vi "_io_read_long_data_chunked_timeout.vi"(4 "Simulation read buffer (\"Simulation\")":string="Simulation", 5 "Timeout for chunked touts (-1: No chunked touts)":i32=-1, 6 "Block Logging (F)":bool, 7 "Block Delay Before Read (F)":bool, 8 "error in":errorcluster caption="error in (no error)", 9 "Trim Response End":bool=TRUE, 10 "Max segment read bytes count (65536)":u32=65536, 11 "VISA resource name":refnum<visa-resource-name>) -> (0 "error out":errorcluster, 1 "TimedOut":bool, 2 "Read buffer":string, 3 "VISA resource name out":refnum<visa-resource-name>)   [LabVIEW 2022 SP3, in "hmp4000_rsidr_core.lvlib"]
doc: "Reads data of unlimited size with chunked VISA timeout - use it for long timeouts, where setting the VISA timeout so high would make the LabVIEW application unresponsive until VISA returns from VISA Read function. The maximum VISA Timeout in this method is 10 seconds, and cumulatively goes up to entered timeout value."
uses:
  hmp4000_rsidr_core.lvlib
  type_Error_Codes.ctl
  type_AdditionalFlag_Bits.ctl
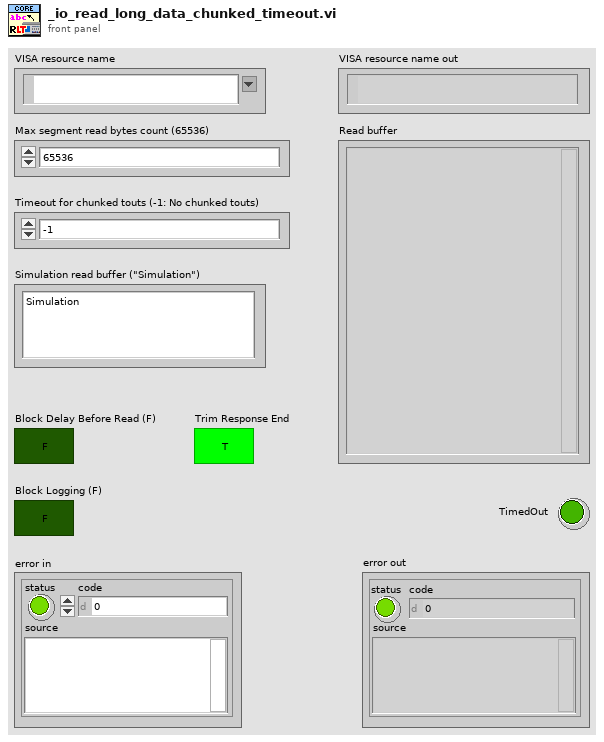
[diagram p1: front panel]
types:
  T1 = typedef "hmp4000_rsidr_core.lvlib/type_AdditionalFlag_Bits.ctl" = enum16{"Send LF after Bin Block", "Junk read with io_clear_buffers.vi", "io_clear_buffers: viClear()", "io_clear_buffers: viFlush()", "<NotUsed1>", "Allow Dbl & Int Bin/Ascii read", "*OPC? in check_instrument_error.vi", "<NotUsed2>", "Smart Enum Matching", "Less Strict RepCaps check", "AssureResponseEndWithLF"}
  T2 = typedef "hmp4000_rsidr_core.lvlib/type_Error_Codes.ctl" = enum16{"No_error", "VISA_err_ResourceNotFound", "VISA_err_Timeout", "VISA_warn_MoreDataAvailable", "RS_err_MissingCallback", "RS_err_InvalidAttribute", "RS_err_InvalidValue", "RS_err_UnknownResource", "RS_err_AlreadyInitialized", "RS_err_InstrumentStatus", "RS_err_BadRepCapName", "RS_err_TypesMismatch", "RS_err_ValueNotSupported", "RS_err_InvalidRngTable", "RS_err_IDqueryFail", "RS_err_UnexpResponse", "VISA_warn_ConfigNotLoaded", "RS_err_AttributeNotReadable", "RS_err_AttributeNotWritable", "RS_err_InstrumentType", "RS_err_InstrumentOption", "VISA_err_InvalidSize", "RS_err_ReliabilityIndicator", "VISA_warn_UnknownStatus", "VISA_warn_TermCharRead", "VISA_err_IO_error", "RS_err_FunctionNotSupported", "VISA_warn_QueueEmpty"}
  T3 = typedef "hmp4000_rsidr_core.lvlib/type_Session_Data.ctl" = cluster{"IDN string":string, "Instrument FW":string, "Instr type":string, "Instr type for err. msg.":string, "Installed Options":string[], "Ignore Error Messages":string, "Logging params":variant, "OPC Timeout":i32, "VISA Timeout":i32, "STB Poll VISA Timeout":i32, "Additional Flags":i32, "Wait Before Read":i32, "Wait Before Write":i32, "Option String Flags":i32, "IO Segment Size":i64, "VISA Access Mode":T4, "Interface Type":T5, "OPC Wait Mode":T6, "Bin Float Number  Format":T7, "Bin Integer Number Format":T8, "Simulate":bool, "VXIcapable":bool, "Duplicate Session":bool, "Add LF to Write":bool, "Logging":bool, "Fast Sweep":bool, "Query Instrument Status":bool, "Check Range":bool, "Check Options":bool}
  T4 = typedef "hmp4000_rsidr_core.lvlib/type_VisaAccessMode.ctl" = u16
  T5 = typedef "hmp4000_rsidr_core.lvlib/type_InterfaceType.ctl" = enum16{"Unknown", "GPIB", "VXI", "GPIB_VXI", "ASRL", "PXI", "TCPIP", "USB", "SOCKET"}
  T6 = typedef "hmp4000_rsidr_core.lvlib/type_OPC_Wait_Mode.ctl" = enum16{"STBpolling", "STBpollingSlow", "STBpollingSuperSlow", "ServiceRequest", "OPCquery"}
  T7 = typedef "hmp4000_rsidr_core.lvlib/type_Binary_Float_Number_Format.ctl" = enum16{"Float_4_Bytes_Swapped", "Float_4_Bytes", "Double_8_Bytes_Swapped", "Double_8_Bytes"}
  T8 = typedef "hmp4000_rsidr_core.lvlib/type_Binary_Integer_Number_Format.ctl" = enum16{"Int32_4_Bytes_Swapped", "Int32_4 Bytes", "Int16_2_Bytes_Swapped", "Int16_2_Bytes"}
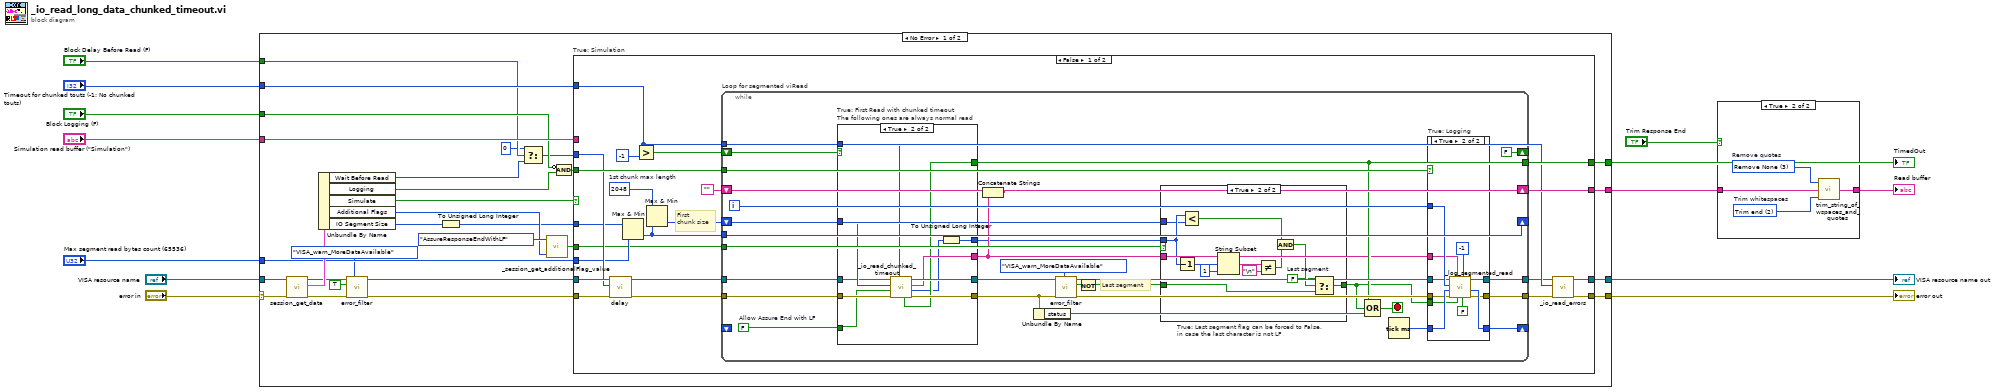
[diagram p0: block diagram]
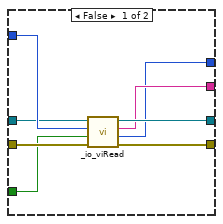
[diagram p5: hidden frame]
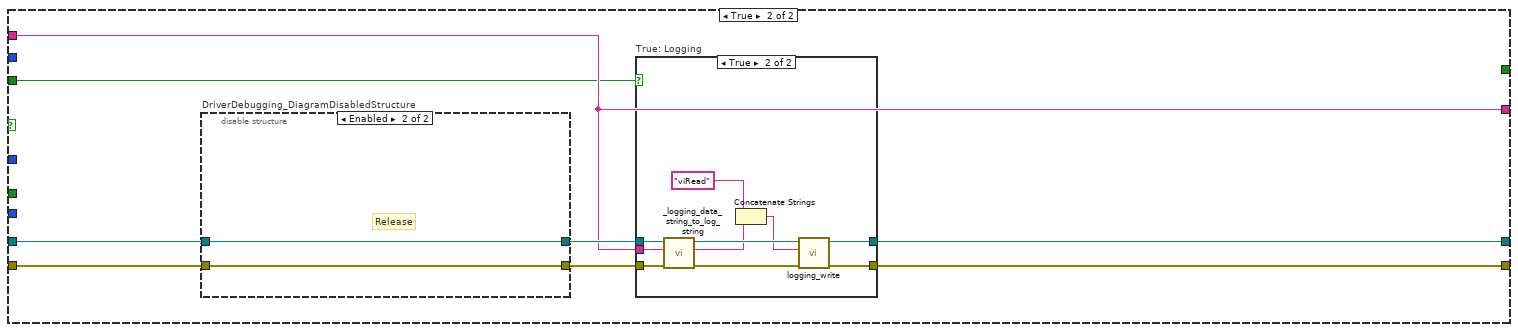
[diagram p6: hidden frame]
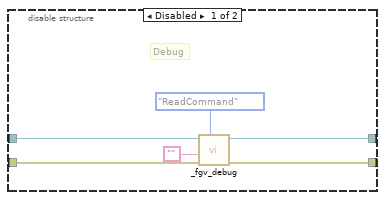
[diagram p8: hidden frame]
diagram:
  n1 = case shown="No Error" "error in" {
    selector: "error in" -> [w42 w171]
    tunnel: [w28 w171] -> w10
    tunnel: "Max segment read bytes count (65536)" -> [w38 _]
    tunnel: [w39 _] -> w2
    tunnel: "VISA resource name" -> [w41 w170]
    tunnel: [w27 w170] -> w9
    tunnel: "Simulation read buffer (\"Simulation\")" -> [w37 _]
    tunnel: "Block Logging (F)" -> [w36 _]
    tunnel: "Timeout for chunked touts (-1: No chunked touts)" -> [w25 _]
    tunnel: [w26 _] -> w5
    tunnel: "Block Delay Before Read (F)" -> [w23 _]
    frame No Error {
      n2 = call "session_get_data.vi"("error in"=w42, "VISA resource name"=w41) -> ("error out"=w35:errorcluster, "Session User Data out"=w40:T3, "VISA resource name out"=w34:refnum<visa-resource-name>)  [unwired: 6 in, 1 out]
      n3 = Unbundle By Name(w40) -> ("Wait Before Read"=w14:i32, "Logging"=w15:bool, "Simulate"=w24:bool, "Additional Flags"=w18:i32, "IO Segment Size"=w17:i64)
      n4 = call "error_filter.vi"("Error Enum in"=type_Error_Codes."VISA_warn_MoreDataAvailable" ("Code to detect"), "error in"=w35, "Clear detected code (F)"=TRUE, "VISA resource name"=w34) -> ("error out"=w31:errorcluster, "VISA resource name out"=w32:refnum<visa-resource-name>)  [unwired: 5 in, 1 out]
      n5 = To Unsigned Long Integer(number=w17) -> (unsigned 32bit integer=w16:u32)
      n6 = Select(t=0, s=w23, f=w14) -> (s? t:f=w22:i32)
      n7 = call "_session_get_additionalFlag_value.vi"("AdditionalFlags value in"=w18, "AdditionalFlag bit"=type_AdditionalFlag_Bits."AssureResponseEndWithLF") -> ("AdditionalFlag bit value out"=w19:bool)  [unwired: 3 in]
      n8 = Compound Arithmetic op=AND(invert w36, w15) -> (w29:bool)
      n9 = case "True: Simulation" shown="False" w24 {
        tunnel: [w58 w144] -> w28
        tunnel: [w59 w145] -> w39
        tunnel: w31 -> [w64 w149]
        tunnel: w32 -> [w63 w148]
        tunnel: [w57 w143] -> w27
        tunnel: w38 -> [w50 _]
        tunnel: w37 -> [_ w145]
        tunnel: w29 -> [w62 w142]
        tunnel: [w56 _] -> w26
        tunnel: w25 -> [w46 _]
        tunnel: w22 -> [w55 _]
        tunnel: w19 -> [w49 _]
        tunnel: w16 -> [w48 _]
        frame False {
          w61 = u32 2048  # 1st chunk max length
          # "First\nchunk size"
          n10 = call "delay.vi"("error in"=w64, "Milliseconds to wait"=w55, "VISA resource name"=w63) -> ("error out"=w54:errorcluster, "VISA resource name out"=w53:refnum<visa-resource-name>)  [unwired: 7 in]
          n11 = Max & Min(x=w48, y=w50) -> (min(x,y)=w52:u32)  [unwired: 1 out]
          n12 = Greater?(x=w46, y=-1) -> (0:w43:bool)
          n13 = Max & Min(x=w61, y=w52) -> (min(x,y)=w51:u32)  [unwired: 1 out]
          n14 = while "Loop for segmented viRead" {
            tunnel: [w94] -> w45
            tunnel: [w93] -> w44
            tunnel: w62 -> [w92]
            tunnel: w53 -> [w90]
            tunnel: w54 -> [w89]
            tunnel: w46 -> [w78]
            shift-right: [w76] -> w59
            shift-left: "" -> [w88]
            shift-right: [w81] -> _
            shift-left: _ -> [_]
            tunnel: [w73] -> w56
            shift-right: [w77] -> _
            shift-left: w51 -> [w65]
            tunnel: w52 -> [w77]
            tunnel: w49 -> [w70]
            shift-right: [FALSE] -> _
            shift-left: w43 -> [w72]
            i -> [w80]
            stop <- w79 stop-if-true
            w75 = FALSE  # Allow Assure End with LF
            # "Last segment"
            n15 = case "True: First Read with chunked timeout\nThe following ones are always normal read" shown="True" w72 {
              tunnel: w90 -> [w128 w139]
              tunnel: [w126 w137] -> w83
              tunnel: w89 -> [w129 w140]
              tunnel: w78 -> [_ w134]
              tunnel: [w125 w136] -> w67
              tunnel: w65 -> [w130 w141]
              tunnel: [w127 w138] -> w82
              tunnel: [_ w135] -> w73
              tunnel: w75 -> [w124 w133]
              tunnel: [w123 w131] -> w66
              frame False {
                n16 = call "_io_viRead.vi"("error in"=w129, "Allow Assure End with LF"=w124, "Max bytes to read"=w130, "VISA resource name"=w128) -> ("error out"=w127:errorcluster, "Read bytes count"=w123:u32, "Read buffer"=w125:string, "VISA resource name out"=w126:refnum<visa-resource-name>)  [unwired: 4 in]
              }
              frame True {
                n17 = call "_io_read_chunked_timeout.vi"("Timeout in"=w134, "error in"=w140, "Allow Assure End with LF"=w133, "Max bytes to read"=w141, "VISA resource name"=w139) -> ("error out"=w138:errorcluster, "Read bytes count"=w132:i32, "Read buffer"=w136:string, "VISA resource name out"=w137:refnum<visa-resource-name>, "TimedOut"=w135:bool)  [unwired: 2 in]
                n18 = To Unsigned Long Integer(number=w132) -> (unsigned 32bit integer=w131:u32)
              }
            }
            n19 = Concatenate Strings(w88, w67) -> (w76:string)
            n20 = Unbundle By Name(w82) -> ("status"=w74:bool)
            n21 = call "error_filter.vi"("Error Enum in"=type_Error_Codes."VISA_warn_MoreDataAvailable" ("Code to detect"), "error in"=w82, "VISA resource name"=w83) -> ("error out"=w86:errorcluster, "Code Detected"=w84:bool, "VISA resource name out"=w85:refnum<visa-resource-name>)  [unwired: 6 in]
            n22 = Not(x=w84) -> (.not. x?=w69:bool)
            n23 = case "True: Last segment flag can be forced to False,\nin case the last character is not LF" shown="True" w70 {
              tunnel: w69 -> [w95 w97]
              tunnel: [w95 w99] -> w68
              tunnel: w67 -> [_ w108]
              tunnel: w66 -> [_ w103]
              tunnel: w65 -> [_ w102]
              frame False {
              }
              frame True {
                w96 = FALSE  # Last segment
                n24 = Decrement(x=w103) -> (x-1=w107:u32)
                n25 = Less?(x=w103, y=w102) -> (x < y?=w100:bool)
                n26 = String Subset(string=w108, offset (0)=w107, length (rest)=1 ("length (rest)")) -> (substring=w105:string)
                n27 = Not Equal?(x=w105, y="\n") -> (x != y?=w101:bool)
                n28 = And(x=w100, y=w101) -> (x .and. y?=w98:bool)
                n29 = Select(t=w96, s=w98, f=w97) -> (s? t:f=w99:bool)
              }
            }
            n30 = Compound Arithmetic op=OR(w73, w68, w74) -> (w79:bool)
            n31 = Tick Count (ms)() -> (millisecond timer value=w91:u32)
            n32 = case "True: Logging" shown="True" w92 {
              tunnel: w86 -> [w111 w118]
              tunnel: [w111 w116] -> w94
              tunnel: w91 -> [w110 w122]
              tunnel: [w110 w121] -> w81
              tunnel: w80 -> [_ w120]
              tunnel: w67 -> [_ w119]
              tunnel: w85 -> [w109 w117]
              tunnel: [w109 w115] -> w93
              tunnel: w68 -> [_ w112]
              frame False {
              }
              frame True {
                n33 = call "_log_segmented_read.vi"("Force binary format (T)"=FALSE, "Total Segments"=-1, "Last Segment"=w112, "Data"=w119, "error in"=w118, "Previous Start Time ms"=w122, "Segment Ix"=w120, "VISA resource name"=w117) -> ("error out"=w116:errorcluster, "New Start Time ms"=w121:u32, "VISA resource name out"=w115:refnum<visa-resource-name>)  [unwired: 1 in]
              }
            }
          }
          n34 = call "_io_read_errors.vi"("error in"=w45, "Custom Timeout (VISA Timeout)"=w46, "VISA resource name"=w44) -> ("error out"=w58:errorcluster, "VISA resource name out"=w57:refnum<visa-resource-name>)  [unwired: 7 in]
        }
        frame True {
          n35 = disable-structure "DriverDebugging_DiagramDisabledStructure" shown="Enabled" {
            disable-tunnel: w149 -> [w166 w168]
            disable-tunnel: [w164 w168] -> w147
            disable-tunnel: w148 -> [w165 w169]
            disable-tunnel: [w163 w169] -> w146
            frame Disabled {
              # "Debug"
              n36 = call "_fgv_debug.vi"("Operation"=enum16{"Reset", "ReadCommand", "SetCommand"}."ReadCommand", "error in"=w166, "Command in"="" ("Empty String Constant"), "VISA resource name"=w165) -> ("error out"=w164:errorcluster, "VISA resource name out"=w163:refnum<visa-resource-name>)  [unwired: 6 in]
            }
            frame Enabled {
              # "Release"
            }
          }
          n37 = case "True: Logging" shown="True" w142 {
            tunnel: w147 -> [w151 w161]
            tunnel: w146 -> [w150 w160]
            tunnel: w145 -> [_ w159]
            tunnel: [w151 w156] -> w144
            tunnel: [w150 w155] -> w143
            frame False {
            }
            frame True {
              n38 = call "_logging_data_string_to_log_string.vi"("error in"=w161, "Raw string to log"=w159, "VISA resource name"=w160) -> ("error out"=w158:errorcluster, "Result log string"=w153:string, "VISA resource name out"=w157:refnum<visa-resource-name>)  [unwired: 6 in]
              n39 = Concatenate Strings("viRead" ("string"), w153) -> (w154:string)
              n40 = call "logging_write.vi"("error in"=w158, "String to write"=w154, "VISA resource name"=w157) -> ("error out"=w156:errorcluster, "VISA resource name out"=w155:refnum<visa-resource-name>)  [unwired: 7 in]
            }
          }
        }
      }
    }
    frame Error {
    }
  }
  "VISA resource name out" <- w9
  "error out" <- w10
  "TimedOut" <- w5
  n41 = case shown="True" "Trim Response End" {
    tunnel: w2 -> [w172 w174]
    tunnel: [w172 w173] -> w1
    frame False {
    }
    frame True {
      w176 = u16 2 items=["Trim both", "Trim start", "Trim end", "Trim none"]  # Trim whitespaces
      w175 = u16 3 items=["Remove All Quotes", "Remove Single Quotes", "Remove Double Quotes", "Remove None"]  # Remove quotes
      n42 = call "trim_string_of_wspaces_and_quotes.vi"("Trim whitespaces (Trim both)"=w176, "String in"=w174, "Remove quotes (Remove All)"=w175) -> ("String out"=w173:string)  [unwired: 2 in]
    }
  }
  "Read buffer" <- w1
